vi "Read Coils Response.vi"(8 "error in (no error)":errorcluster, 9 "Modbus Data Unit in":T1={"function"=1, "Data"=[]} {"function" items=["Read Discrete Inputs"=2, "Read Coils"=1, "Write Single Coil"=5, "Write Multiple Coils"=15, "Read Input Register"=4, "Read Holding Registers"=3, "Write Single Register"=6, "Write Multiple Registers"=16, "Read/Write Multiple Registers"=23, "Mask Write Register"=22, "Read FIFO Queue"=24, "Read File Record"=20, "Write File Record"=21, "Read Exception Status"=7, "Diagnostic"=8, "Get Com Event Counter"=11, "Get Com Event Log"=12, "Report Slave ID"=17, "Read Device Identification"=43]; "Data" format="%.0x"}) -> (0 "error out":errorcluster, 2 "data":bool[](array[boolean]))   [LabVIEW 2021, in "NI_modbus_upd.lvlib"]
doc: "Decodes the response for the read coils function."
uses:
  NI_modbus_upd.lvlib
  Ctl/MB Modbus Data Unit.ctl
  Modbus Data Unit (PDU)/Function.ctl
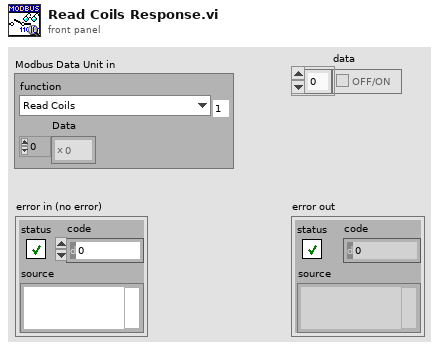
[diagram p1: front panel]
types:
  T1 = typedef "NI_modbus_upd.lvlib/MB Modbus Data Unit.ctl" = cluster{"function":T2, "Data":u8[]}
  T2 = typedef "NI_modbus_upd.lvlib/Function.ctl" = u8
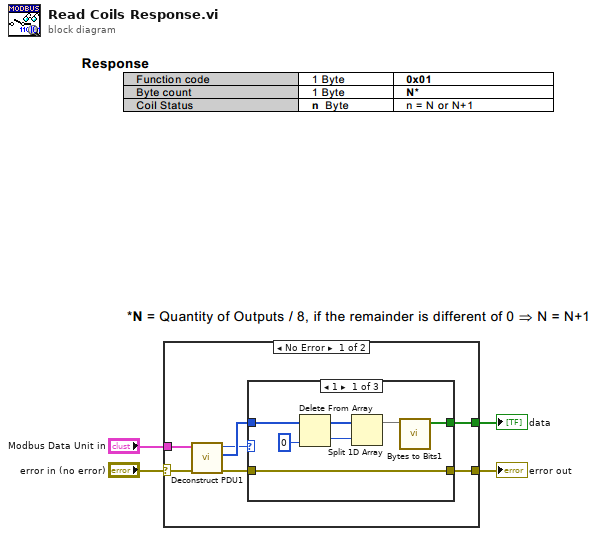
[diagram p0: block diagram]
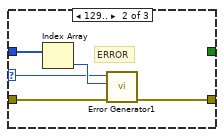
[diagram p2: hidden frame]
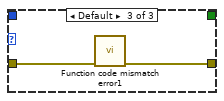
[diagram p3: hidden frame]
diagram:
  n1 = case shown="No Error" "error in (no error)" {
    selector: "error in (no error)" -> [w7 w26]
    tunnel: [w11 w26] -> w4
    tunnel: "Modbus Data Unit in" -> [w6 _]
    tunnel: [w10 _] -> w3
    frame No Error {
      n2 = call "Deconstruct PDU1.vi"("error in (no error)"=w7, "Modbus Data Unit in"=w6) -> ("error out"=w8:errorcluster, "data"=w9:u8[], "function"=w5:T2)  [unwired: 7 in]
      n3 = case shown="1" w5 {
        selector: w5 -> [_ w19 _]
        tunnel: w8 -> [w16 w20 w25]
        tunnel: w9 -> [w18 w23 _]
        tunnel: [w16 w22 w24] -> w11
        tunnel: [w17 _ _] -> w10
        frame 1 {
          n4 = Delete From Array(array=w18, index=0) -> (deleted portion=w14:u8, array with subset deleted=w13:u8[])  [unwired: 1 in]
          n5 = Split 1D Array(array=w13, index=w14) -> (first subarray=w15:u8[])  [unwired: 1 out]
          n6 = call "Bytes to Bits1.vi"("bytes"=w15) -> ("bits"=w17:bool[])  [unwired: 10 in]
        }
        frame 129.. {
          # "ERROR"
          n7 = Index Array(array=w23) -> (element=w21:u8)  [unwired: 1 in]
          n8 = call "Error Generator1.vi"("error in (no error)"=w20, "data return (error code)"=w21, "function return"=w19) -> ("error out"=w22:errorcluster)  [unwired: 8 in]
        }
        frame Default {
          n9 = call "Function code mismatch error1.vi"("error in (no error)"=w25) -> ("error out"=w24:errorcluster)  [unwired: 10 in]
        }
      }
    }
    frame Error {
    }
  }
  "error out" <- w4
  "data" <- w3
